vi "EnableWFGOutput.vi"(0 "object in":refnum<class "AD2_SDK.lvclass">, 2 "OutputEnable 2":T1, 5 "error in (no error)":errorcluster) -> (14 "object out":refnum<class "AD2_SDK.lvclass">, 19 "error out":errorcluster)   [LabVIEW 2019, in "AD2_SDK.lvclass"]
uses:
  AD2_SDK.lvclass
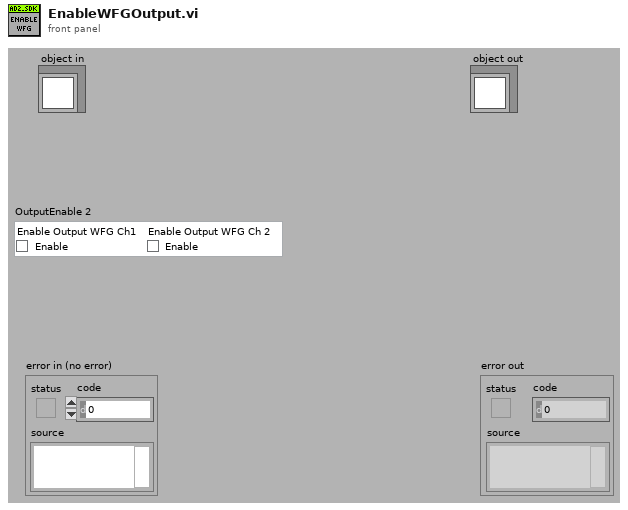
[diagram p1: front panel]
types:
  T1 = cluster{"Enable Output WFG Ch1":bool, "Enable Output WFG Ch 2":bool}
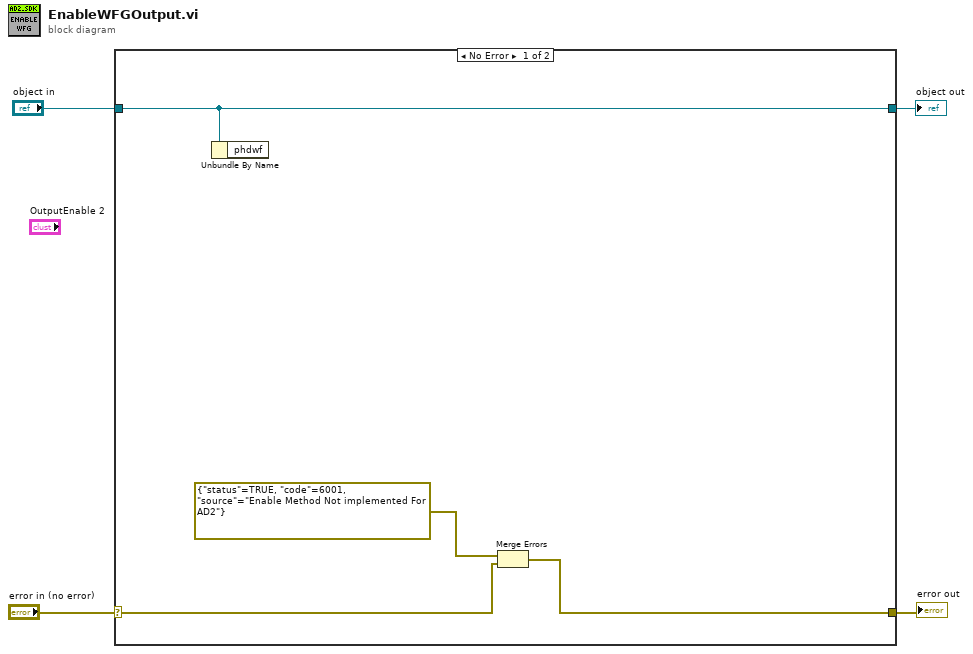
[diagram p0: block diagram]
diagram:
  n1 = case shown="No Error" "error in (no error)" {
    selector: "error in (no error)" -> [w6 w10]
    tunnel: [w5 w10] -> w3
    tunnel: [w8 w9] -> w1
    tunnel: "object in" -> [w8 w9]
    frame No Error {
      n2 = Unbundle By Name(w8) -> ()  [unwired: 1 out]
      n3 = Merge Errors(errorcluster {"status"=TRUE, "code"=6001, "source"="Enable Method Not implemented For AD2"} ("error in (no error)"), w6) -> (w5:errorcluster)
    }
    frame Error {
    }
  }
  "error out" <- w3
  "object out" <- w1
